vi "Send-heartbeat.vi"(8 "error in (no error)":errorcluster, 11 "Client in":T1) -> (0 "error out":errorcluster, 3 "Client out":T1)   [LabVIEW 2013, in "PowderDeposition.lvlib" / "PD-Client.lvclass"]
doc: "Wrapper function for sending the specific 'Hearbeat' type message.\nThis function creates and immediately sends a heartbeat message to the server, using the configuration of the client object."
uses:
  PD-Client.lvclass
  Object-reference.ctl
  PD-Client.lvclass/PD-Client.ctl
  SA-SLMAPI/Sources/Heartbeat/Heartbeat.lvclass
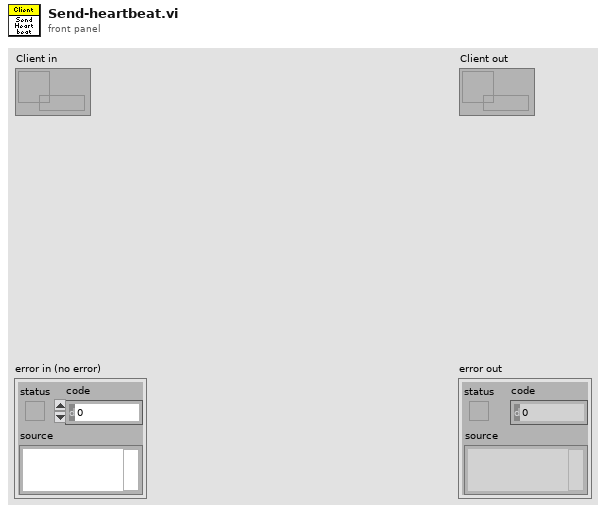
[diagram p1: front panel]
types:
  T1 = typedef "PowderDeposition.lvlib/PD-Client.lvclass/Object-reference.ctl" = refnum<data-value>
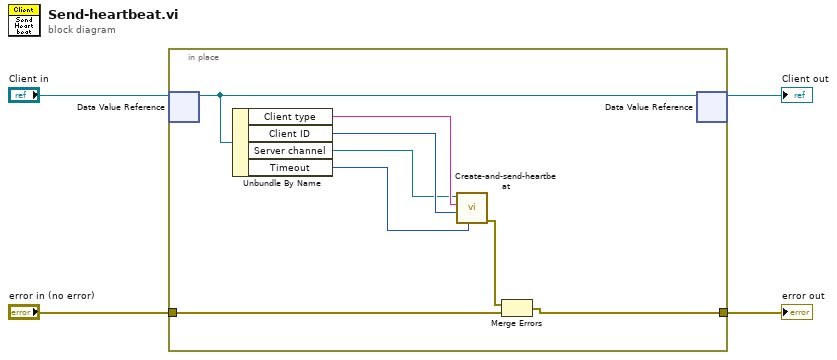
[diagram p0: block diagram]
diagram:
  n1 = in-place {
    in-place-border: "error in (no error)" -> [w6]
    in-place-border: [w5] -> w3
    n2 = in-place-dvr #1("Client in") -> (w8:refnum<class "PD-Client.lvclass">)  [unwired: 1 out]
    n3 = Unbundle By Name(w8) -> ("Client type"=w12:string, "Client ID"=w11:i32, "Server channel"=w10:refnum<queue>, "Timeout"=w9:i32)
    n4 = call "Create-and-send-heartbeat.vi"("Timeout"=w9, "Sender ID"=w11, "Sender"=w12, "Server channel"=w10) -> ("error out"=w7:errorcluster)  [unwired: 7 in]
    n5 = Merge Errors(w7, w6) -> (w5:errorcluster)
    n6 = in-place-dvr #1(w8) -> (→"Client out":T1)  [unwired: 1 out]
  }
  "error out" <- w3
